vi "Read Devices.vi"(11 "Test Framework in":refnum<class "Test Framework.lvclass">) -> (2 "Devices":refnum<class "Device.lvclass">[](array[class]), 3 "Test Framework out":refnum<class "Test Framework.lvclass">)   [LabVIEW 2020, in "Test Framework.lvclass"]
uses:
  Test Framework.lvclass
  Devices/Device.lvclass
  Test Framework.lvclass/Test Framework.ctl
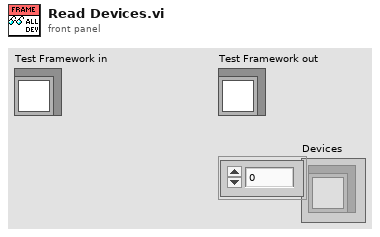
[diagram p1: front panel]
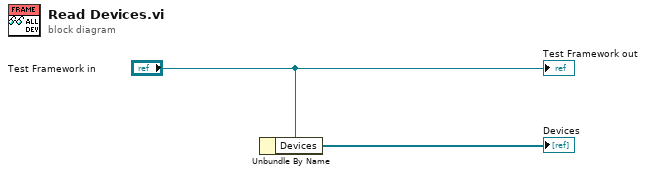
[diagram p0: block diagram]
diagram:
  n1 = Unbundle By Name("Test Framework in") -> ("Devices"=→"Devices":refnum<class "Device.lvclass">[])
  "Test Framework out" <- "Test Framework in"
